vi "批量设置.vi"() -> (2 "启动命令 2":T1 caption="启动命令", 3 "确定 2":bool)   [LabVIEW 2016, in "ZK定时设置.xctl"]
uses:
  <vilib>/Utility/miscctls.llb/LVPointTypeDef.ctl
panel:
  in  "取消":bool
  in  "确定":bool
  in  "启动命令":T1 caption="启动模式"
  # "请选择批量设置模式"
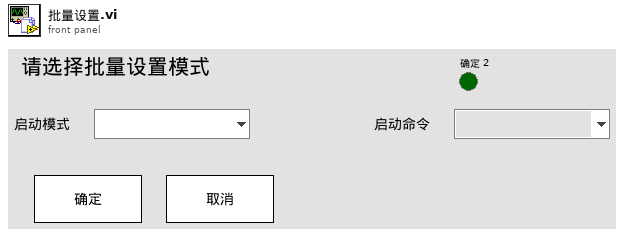
[diagram p1: front panel]
types:
  T1 = typedef "ZK定时设置.xctl/启动命令选择.ctl" = enum16{"", "加标回收（启动采配水）", "加标回收（不启动采配水）", "水样测试（启动采配水）", "水样测试（不启动采配水）", "平行样测试（启动采配水）", "平行样测试（不启动采配水）", "集成干预测试"}
  T2 = typedef "LVPointTypeDef.ctl" = cluster{"Horizontal":i16, "Vertical":i16}
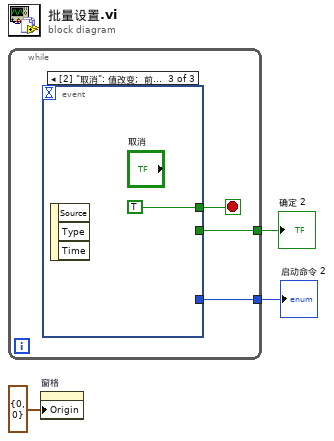
[diagram p0: block diagram]
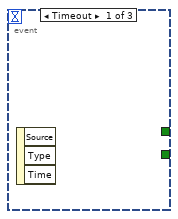
[diagram p2: hidden frame]
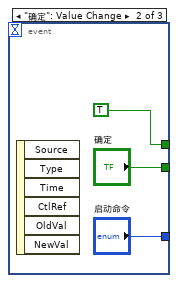
[diagram p3: hidden frame]
diagram:
  n1 = while {
    tunnel: [w6] -> w3
    tunnel: [w5] -> w1
    stop <- w4 stop-if-true
    n2 = event shown="[2] \"取消\": 值改变;  前面板关闭" {
      selector: _ -> [_ _ _]
      dyn-events: _ -> [_ _ _]
      timeout: _ -> [_ _ _]
      tunnel: [_ "启动命令" _] -> w6
      tunnel: [_ "确定" _] -> w5
      tunnel: [_ TRUE TRUE] -> w4
      event Timeout {
        n3 = event-data() -> ()  [unwired: 1 in, 3 out]
      }
      event "确定": Value Change {
        n4 = event-data() -> ()  [unwired: 1 in, 6 out]
      }
      event "取消": Value Change; Panel Close {
        n5 = event-data() -> ()  [unwired: 1 in, 3 out]
      }
    }
  }
  "启动命令 2" <- w3
  "确定 2" <- w1
  n6 = property on="窗格" class="Pane"("Origin"=T2 {"Horizontal"=0, "Vertical"=0} ("原点")) -> ()  [unwired: 2 in, 2 out]
